vi "FTW-JSON-SerializeElement.vi"(0 "JSON":refnum<class "FTW-Container.lvclass">, 5 "Key":string, 11 "error in":errorcluster) -> (4 "JSON out":refnum<class "FTW-Container.lvclass">, 6 "Element as JSON String":string, 10 "Found?":bool, 15 "error out":errorcluster)   [LabVIEW 2015]
uses:
  container/FTW-Container.lvclass
panel:
  # "Inputs"
  # "Outputs"
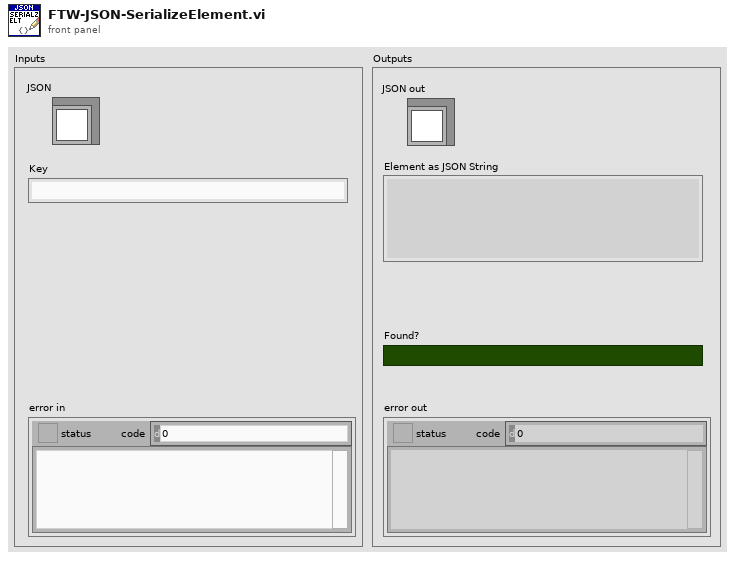
[diagram p1: front panel]
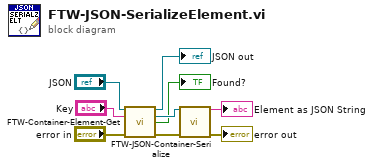
[diagram p0: block diagram]
diagram:
  n1 = call "FTW-Container-Element-Get.vi"("FTW-Container In"="JSON", "Element Name"="Key", "error in"="error in") -> ("FTW-Container Out"=→"JSON out":refnum<class "FTW-Container.lvclass">, "Element Out"=w3:refnum<class "FTW-Container.lvclass">, "Found"=→"Found?":bool, "error out"=w8:errorcluster)  [unwired: 9 in]
  n2 = call "FTW-JSON-Container-Serialize.vi"("Container"=w3, "error in"=w8) -> ("JSON String"=→"Element as JSON String":string, "error out"=→"error out":errorcluster)  [unwired: 12 in]
